vi "CalcJacobian.vi"(7 "EndEff Velocities":T1=[[0.0], [0.0]], 8 "q2":dbl, 9 "q1":dbl, 10 "L2":dbl, 11 "L1":dbl) -> (2 "Joint Angular Velocities":T1, 3 "Jacobian":dbl[][](array[numeric]))   [LabVIEW 2024]
uses:
  <vilib>/Analysis/Matrix/Datatypes/RealMatrix.ctl
  <vilib>/Analysis/_algsub.llb/Real PseudoInverse Matrix.vi
  <vilib>/Analysis/baseanly.llb/Real A x B.vi
  <vilib>/Analysis/NI_AALPro.lvlib
  <vilib>/Analysis/NI_AALBase.lvlib
  <vilib>/Analysis/Matrix/NI_Matrix.lvlib
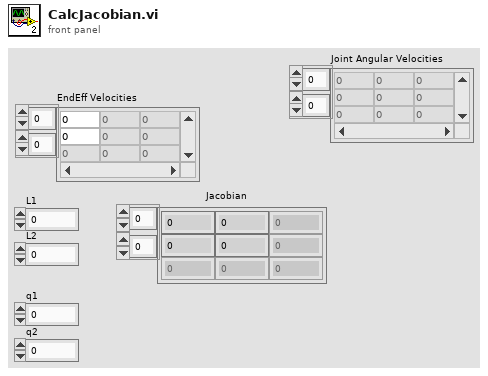
[diagram p1: front panel]
types:
  T1 = typedef "NI_Matrix.lvlib/RealMatrix.ctl" = dbl[][]
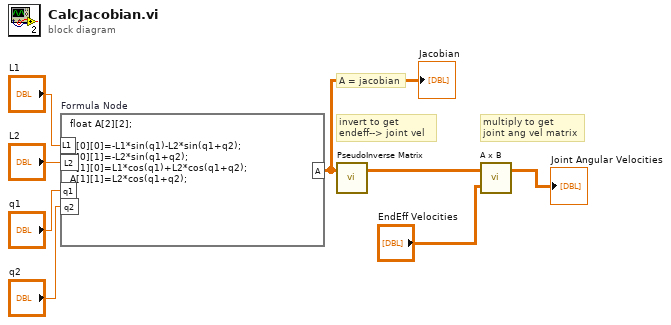
[diagram p0: block diagram]
diagram:
  # "multiply to get\njoint ang vel matrix"
  # "invert to get \nendeff--> joint vel"
  # "A = jacobian"
  n1 = formula code="float A[2][2];\n\nA[0][0]=-L1*sin(q1)-L2*sin(q1+q2);\nA[0][1]=-L2*sin(q1+q2);\nA[1][0]=L1*cos(q1)+L2*cos(q1+q2);\nA[1][1]=L2*cos(q1+q2);"("L1"="L1", "L2"="L2", "q1"="q1", "q2"="q2") -> ("A"=w4:dbl[][])
  "Jacobian" <- w4
  n2 = call-poly <vilib>:"PseudoInverse Matrix.vi"("Input Matrix"=w4) -> ("PseudoInverse Matrix"=w3:T1)  [unwired: 1 in, 1 out]
  n3 = call-poly <vilib>:"A x B.vi"("B"="EndEff Velocities", "A"=w3) -> ("A x B"=→"Joint Angular Velocities":T1)  [unwired: 1 out]
